vi "VST Streaming.vi"() -> ()   [LabVIEW 2021]
doc: "Demonstrates how to acquire I/Q data using the RF vector signal analyzer. The example shows how to configure NI-RFSA for continuous I/Q acquisition, how to set the carrier frequency and the I/Q rate, and how to fetch I/Q data. The dBm calculation is applied to I/Q magnitude to produce signal power and display it on the graph."
uses:
  Messaging/Write Message with Waveform.ctl
  RFSA/Support/RFSA Configuration.ctl
  Messaging/RFSA Message.ctl
  RFSG/Support/RFSG Configuration.ctl
  Messaging/RFSG Message.ctl
panel:
  in  "bandwidth":dbl(slide)=1000000.0 caption="Bandwidth" min=10000.0 max=200000000.0 step=1000000.0 scale=10000.0..200000000.0
  in  "freq.off":i32(slide)=2 caption="Frequency Offset" min=0 max=10000000 step=1000 scale=0.0..10000000.0 scale format="%.0pHz"
  in  "resolution":i64(slide)=1000 caption="Resolution" min=1000 max=100000 step=1000 scale=100000.0..1000.0
  in  "center.freq":dbl(slide)=4000000000.0 caption="Center Frequency" min=500000000.0 max=5500000000.0 step=500000000.0 scale=500000000.0..5500000000.0 scale format="%.1f"
  in  "pwr":dbl(slide)=-10.0 caption="Power" min=-60.0 max=0.0 step=1.0
  in  "rfsg.rsrc":refnum<k15>="5646VST" caption="RFSG Resource"
  in  "rfsa.rsrc":refnum<k15>="5646VST" caption="RFSA Resource"
  in  "start.rf":bool
  in  "stop.rf":bool
  in  "write?":bool
  in  "plot iq?":bool
  out "pred.acq.rate":dbl caption="Predicted Acquisition Rate" format="%#_4pB/s"
  out "pred.blk.size":dbl caption="Predicted Block Size" format="%#_4pB"
  in  "Clear Charts":bool
  out "Write to Disk Rate":dbl format="%#_4pB/s"
  out "Actual Execution Rate":dbl format="%#_4pB/s"
  out "Actual Acquisition Rate":dbl format="%#_4pB/s"
  out "Actual Block Size":i32 format="%.0pB"
  out "iq data":cluster{dbl[], dbl[]}(graph)
  # "200MHz"
  # "10kHz"
  # "10MHz"
  # "0Hz"
  # "1kHz"
  # "100kHz"
  # "5.5GHz"
  # "500MHz"
  # "0dB"
  # "-60dB"
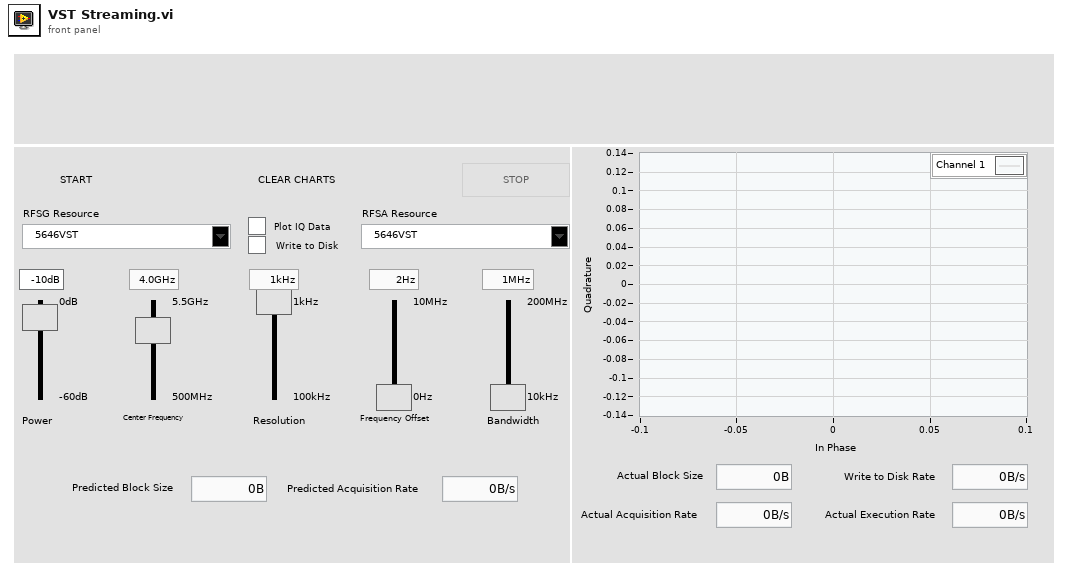
[diagram p1: front panel]
types:
  T1 = enum8{"Enabled", "Disabled", "Disabled and Grayed Out"}
  T2 = typedef "RFSG Configuration.ctl" = cluster{"rfsg ref":refnum<k15>, "freq off":i32, "wfm type":u16, "cent freq":dbl, "iq rate":dbl, "power":dbl, "msg":T3}
  T3 = typedef "RFSG Message.ctl" = enum16{"Trigger Ready", "Run RF", "Stop RF", "Exit"}
  T4 = typedef "RFSA Configuration.ctl" = cluster{"rfsa ref":refnum<k15>, "cent freq":dbl, "iq rate":dbl, "power":dbl, "N/block":i64, "msg":T5}
  T5 = typedef "RFSA Message.ctl" = enum16{"Trigger Ready", "Run RF", "Stop RF", "Exit"}
  T6 = typedef "Write Message with Waveform.ctl" = cluster{"wfm dat":waveform(cdb), "msg":enum16{"Close TDMS", "Initialize TDMS", "Write", "Exit"}}
  T7 = enum32{"invalid app kind", "Development System", "Run Time System", "Student Edition", "Embedded LabVIEW", "Evaluation", "Custom"}
  T8 = enum16{"Close TDMS", "Initialize TDMS", "Write", "Exit"}
  T9 = enum16{"open", "open or create", "create or replace", "create", "open (read-only)"}
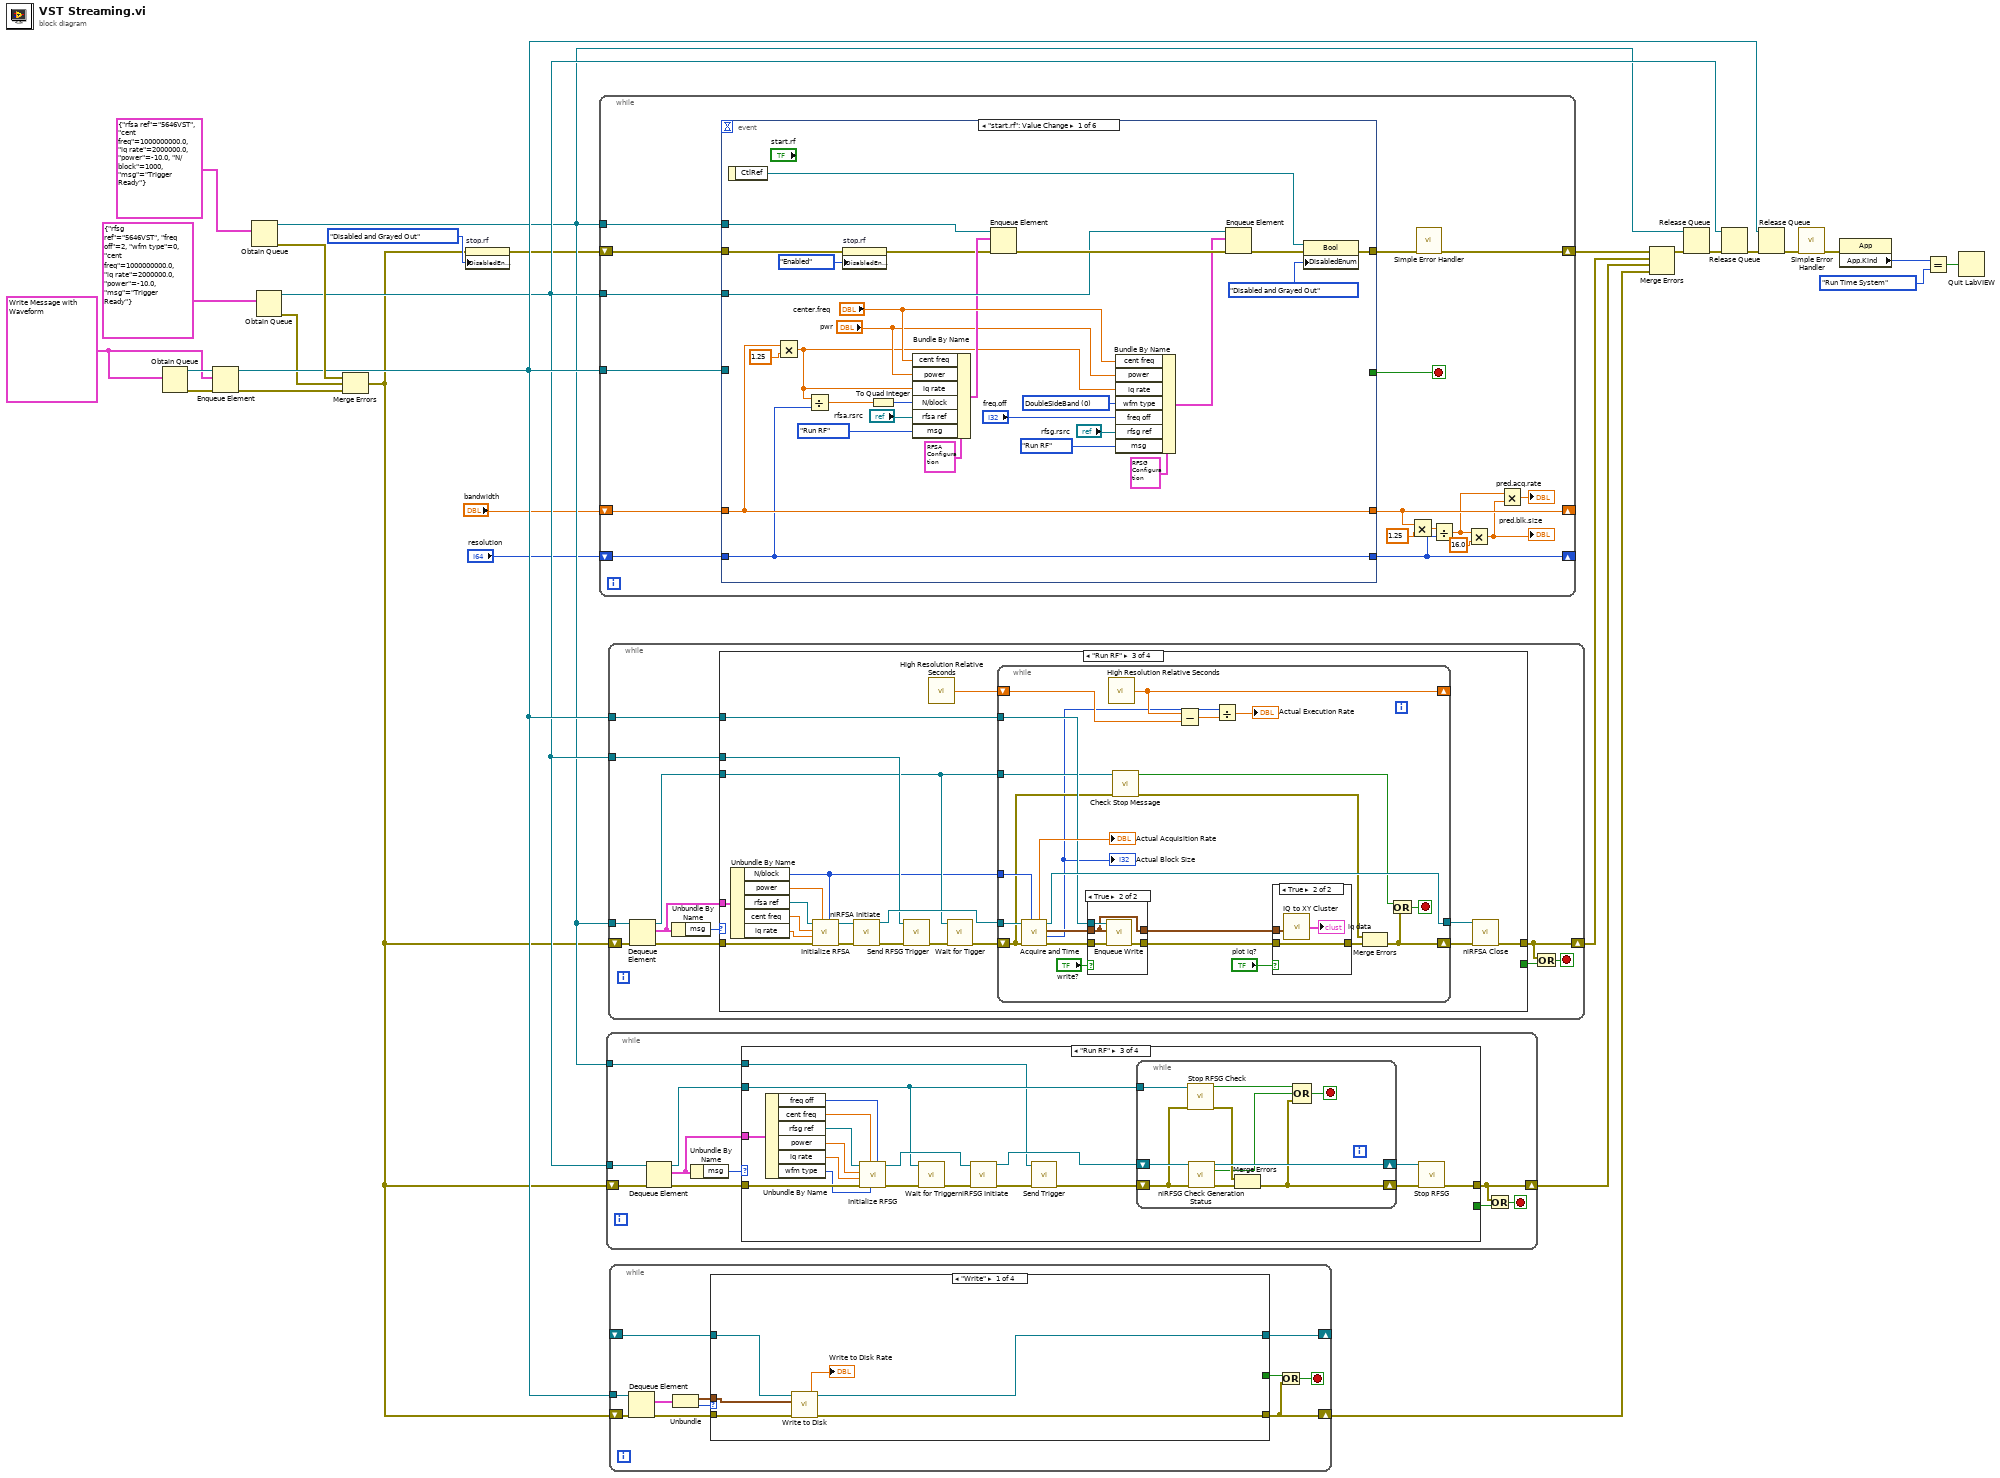
[diagram p0: block diagram]
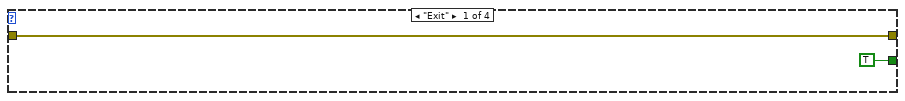
[diagram p2: hidden frame]
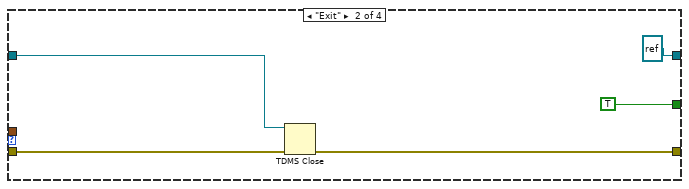
[diagram p5: hidden frame]
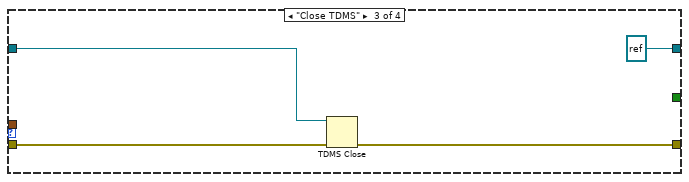
[diagram p6: hidden frame]
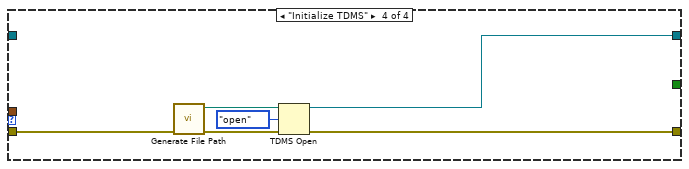
[diagram p7: hidden frame]
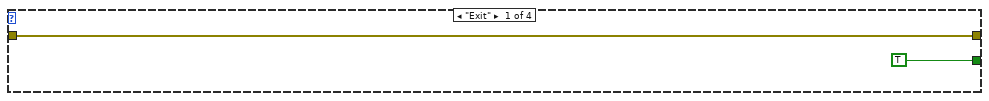
[diagram p8: hidden frame]
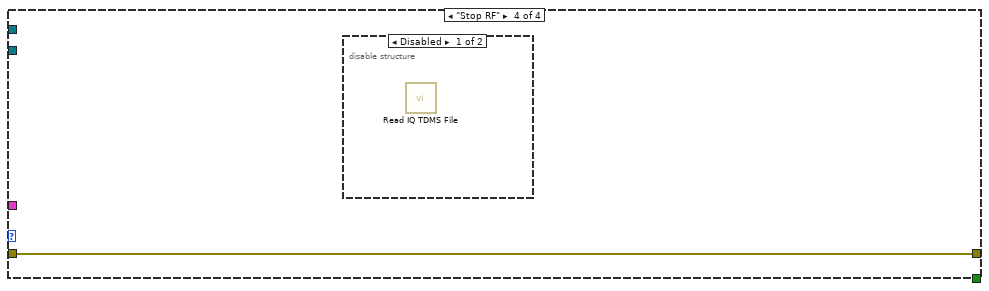
[diagram p12: hidden frame]
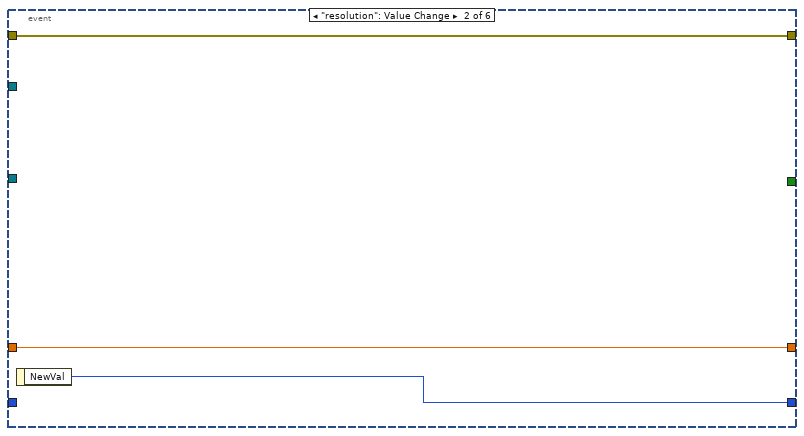
[diagram p14: hidden frame]
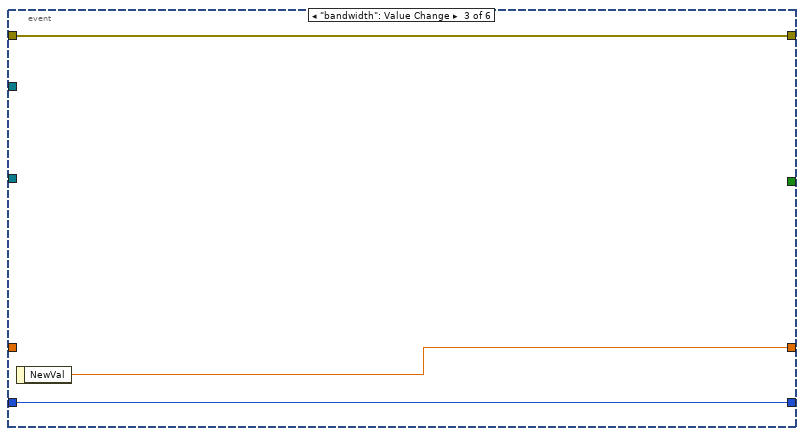
[diagram p15: hidden frame]
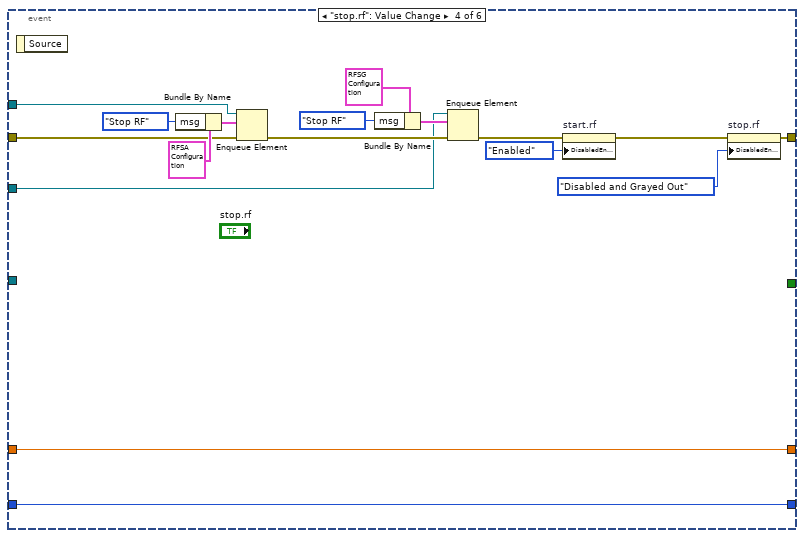
[diagram p16: hidden frame]
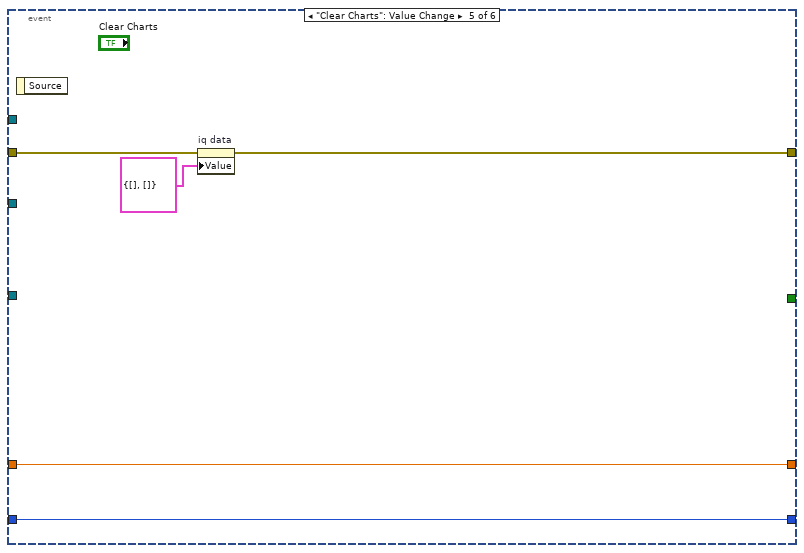
[diagram p17: hidden frame]
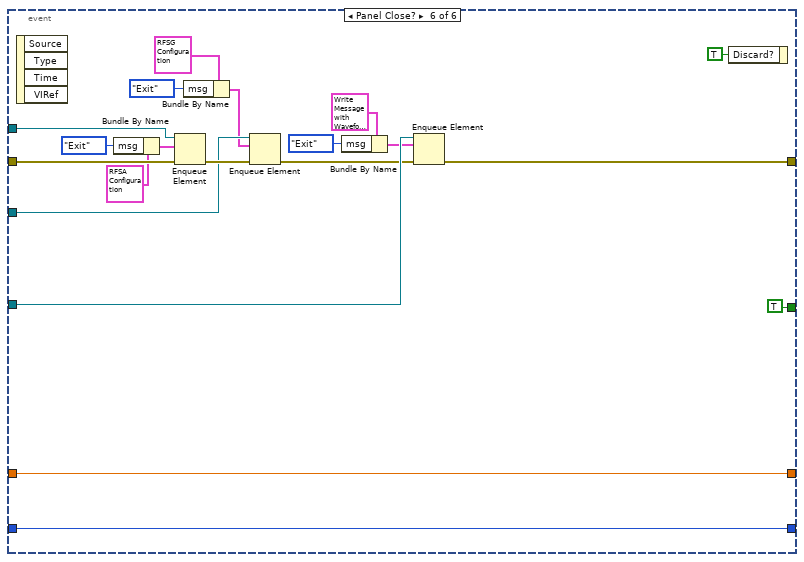
[diagram p18: hidden frame]
diagram:
  w18 = T6 {"wfm dat"={"t0"=timestamp(0 s since 1904-01-01), "dt"=0.0, "Y"=[]}, "msg"=enum."Initialize TDMS"}
  n1 = Obtain Queue(element data type=w18) -> (queue out=w24:refnum<queue>, error out=w25:errorcluster)  [unwired: 4 in, 1 out]
  n2 = Enqueue Element(queue=w24, element=w18, error in (no error)=w25) -> (queue out=w17:refnum<queue>, error out=w14:errorcluster)  [unwired: 1 in, 1 out]
  n3 = Obtain Queue(element data type=T4 {"rfsa ref"="5646VST", "cent freq"=1000000000.0, "iq rate"=2000000.0, "power"=-10.0, "N/block"=1000, "msg"=enum."Trigger Ready"}) -> (queue out=w7:refnum<queue>, error out=w19:errorcluster)  [unwired: 4 in, 1 out]
  n4 = Obtain Queue(element data type=T2 {"rfsg ref"="5646VST", "freq off"=2, "wfm type"=0, "cent freq"=1000000000.0, "iq rate"=2000000.0, "power"=-10.0, "msg"=enum."Trigger Ready"}) -> (queue out=w8:refnum<queue>, error out=w13:errorcluster)  [unwired: 4 in, 1 out]
  n5 = Merge Errors(w19, w13, w14) -> (w4:errorcluster)
  n6 = property on="stop.rf" class="Bool"(error in=w4, "DisabledEnum"=T1."Disabled and Grayed Out" ("Disabled")) -> (error out=w3:errorcluster)  [unwired: 1 in, 1 out]
  n7 = while {
    shift-right: [w32] -> w28
    shift-left: w3 -> [w44]
    tunnel: w7 -> [w45]
    tunnel: w17 -> [w43]
    tunnel: w8 -> [w42]
    shift-right: [w31] -> _
    shift-left: "bandwidth" -> [w39]
    shift-right: [w35] -> _
    shift-left: "resolution" -> [w38]
    stop <- w34 stop-if-true
    n8 = event shown="[0] \"start.rf\": Value Change" {
      selector: _ -> [_ _ _ _ _ _]
      dyn-events: _ -> [_ _ _ _ _ _]
      timeout: _ -> [_ _ _ _ _ _]
      tunnel: w45 -> [w73 _ _ w88 _ w120]
      tunnel: w44 -> [w52 w74 w77 w89 w101 w121]
      tunnel: [w71 w74 w77 w83 w100 w104] -> w33
      tunnel: [_ _ _ _ _ TRUE ("Exit")] -> w34
      tunnel: w43 -> [_ _ _ _ _ w118]
      tunnel: w42 -> [w66 _ _ w87 _ w108]
      tunnel: w39 -> [w47 w75 _ w80 w98 w103]
      tunnel: [w46 w76 w78 w81 w97 w102] -> w35
      tunnel: w38 -> [w46 _ w78 w81 w97 w102]
      tunnel: [w47 w75 w79 w80 w98 w103] -> w31
      event "start.rf": Value Change {
        w62 = u16 0 items=["DoubleSideBand", "LowerSideBand", "UpperSideBand"] ("Selected Waveform")
        n9 = event-data() -> ("CtlRef"=w70:refnum<vi>)  [unwired: 1 in]
        n10 = Multiply(x=w47, y=1.25) -> (x*y=w49:dbl)
        n11 = Divide(x=w49, y=w46) -> (x/y=w56:dbl)
        n12 = property on="stop.rf" class="Bool"(error in=w52, "DisabledEnum"=T1."Enabled" ("Disabled")) -> (error out=w51:errorcluster)  [unwired: 1 in, 1 out]
        n13 = To Quad Integer(1:w56) -> (0:w48:i64)
        n14 = Bundle By Name(cluster=T4 {"rfsa ref"="5646VST", "cent freq"=1000000000.0, "iq rate"=2000000.0, "power"=-10.0, "N/block"=1000, "msg"=enum."Trigger Ready"} ("element"), "cent freq"="center.freq", "power"="pwr", "iq rate"=w49, "N/block"=w48, "rfsa ref"="rfsa.rsrc", "msg"=RFSA_Message."Run RF") -> (w59:T4)
        n15 = Enqueue Element(queue=w73, element=w59, error in (no error)=w51) -> (error out=w68:errorcluster)  [unwired: 1 in, 2 out]
        n16 = Bundle By Name(cluster=T2 {"rfsg ref"="5646VST", "freq off"=2, "wfm type"=0, "cent freq"=1000000000.0, "iq rate"=2000000.0, "power"=-10.0, "msg"=enum."Trigger Ready"} ("element"), "cent freq"="center.freq", "power"="pwr", "iq rate"=w49, "wfm type"=w62, "freq off"="freq.off", "rfsg ref"="rfsg.rsrc", "msg"=RFSG_Message."Run RF") -> (w57:T2)
        n17 = Enqueue Element(queue=w66, element=w57, error in (no error)=w68) -> (error out=w67:errorcluster)  [unwired: 1 in, 2 out]
        n18 = property class="Bool"(reference=w70, error in=w67, "DisabledEnum"=T1."Disabled and Grayed Out" ("Disabled")) -> (error out=w71:errorcluster)  [unwired: 1 out]
      }
      event "resolution": Value Change {
        n19 = event-data() -> ("NewVal"=w76:i64)  [unwired: 1 in]
      }
      event "bandwidth": Value Change {
        n20 = event-data() -> ("NewVal"=w79:dbl)  [unwired: 1 in]
      }
      event "stop.rf": Value Change {
        n21 = event-data() -> ()  [unwired: 1 in, 1 out]
        n22 = Bundle By Name(cluster=T4 {"rfsa ref"="5646VST", "cent freq"=1000000000.0, "iq rate"=2000000.0, "power"=-10.0, "N/block"=1000, "msg"=enum."Trigger Ready"} ("element"), "msg"=RFSA_Message."Stop RF") -> (w94:T4)
        n23 = Enqueue Element(queue=w88, element=w94, error in (no error)=w89) -> (error out=w93:errorcluster)  [unwired: 1 in, 2 out]
        n24 = Bundle By Name(cluster=T2 {"rfsg ref"="5646VST", "freq off"=2, "wfm type"=0, "cent freq"=1000000000.0, "iq rate"=2000000.0, "power"=-10.0, "msg"=enum."Trigger Ready"} ("element"), "msg"=RFSG_Message."Stop RF") -> (w90:T2)
        n25 = Enqueue Element(queue=w87, element=w90, error in (no error)=w93) -> (error out=w86:errorcluster)  [unwired: 1 in, 2 out]
        n26 = property on="start.rf" class="Bool"(error in=w86, "DisabledEnum"=T1."Enabled" ("Disabled")) -> (error out=w84:errorcluster)  [unwired: 1 in, 1 out]
        n27 = property on="stop.rf" class="Bool"(error in=w84, "DisabledEnum"=T1."Disabled and Grayed Out" ("Disabled")) -> (error out=w83:errorcluster)  [unwired: 1 in, 1 out]
      }
      event "Clear Charts": Value Change {
        n28 = event-data() -> ()  [unwired: 1 in, 1 out]
        n29 = property on="iq data" class="XYGraph (strict)"(error in=w101, "Value"=cluster{dbl[], dbl[]} {[], []} ("iq data")) -> (error out=w100:errorcluster)  [unwired: 1 in, 1 out]
      }
      event Panel Close? {
        n30 = event-data() -> ()  [unwired: 1 in, 4 out]
        n31 = Bundle By Name(cluster=T4 {"rfsa ref"="5646VST", "cent freq"=1000000000.0, "iq rate"=2000000.0, "power"=-10.0, "N/block"=1000, "msg"=enum."Trigger Ready"} ("element"), "msg"=RFSA_Message."Exit") -> (w111:T4)
        n32 = Enqueue Element(queue=w120, element=w111, error in (no error)=w121) -> (error out=w110:errorcluster)  [unwired: 1 in, 2 out]
        n33 = Bundle By Name(cluster=T2 {"rfsg ref"="5646VST", "freq off"=2, "wfm type"=0, "cent freq"=1000000000.0, "iq rate"=2000000.0, "power"=-10.0, "msg"=enum."Trigger Ready"} ("element"), "msg"=RFSG_Message."Exit") -> (w105:T2)
        n34 = Enqueue Element(queue=w108, element=w105, error in (no error)=w110) -> (error out=w109:errorcluster)  [unwired: 1 in, 2 out]
        n35 = Bundle By Name(cluster=T6 {"wfm dat"={"t0"=timestamp(0 s since 1904-01-01), "dt"=0.0, "Y"=[]}, "msg"=enum."Exit"} ("element"), "msg"=T8."Exit") -> (w115:T6)
        n36 = Enqueue Element(queue=w118, element=w115, error in (no error)=w109) -> (error out=w104:errorcluster)  [unwired: 1 in, 2 out]
        n37 = event-data("Discard?"=TRUE) -> ()  [unwired: 1 in, 1 out]
      }
    }
    n38 = Multiply(x=w31, y=1.25) -> (x*y=w36:dbl)
    n39 = call <vilib>:"Simple Error Handler.vi"("error in (no error)"=w33) -> ("error out"=w32:errorcluster)  [unwired: 4 in, 4 out]
    n40 = Divide(x=w36, y=w35) -> (x/y=w29:dbl)
    n41 = Multiply(x=w29, y=16.0) -> (x*y=w30:dbl)
    "pred.blk.size" <- w30
    n42 = Multiply(x=w29, y=w30) -> (x*y=→"pred.acq.rate":dbl)
  }
  n43 = while {
    shift-right: [w127] -> w9
    shift-left: w4 -> [w130]
    tunnel: w8 -> [w126]
    tunnel: w7 -> [w122]
    stop <- w129 stop-if-true
    n44 = Dequeue Element(queue=w126, error in (no error)=w130) -> (queue out=w123:refnum<queue>, element=w125:T2, error out=w131:errorcluster)  [unwired: 1 in, 1 out]
    n45 = Unbundle By Name(w125) -> ("msg"=w124:T3)
    n46 = case shown="\"Run RF\"" w124 {
      tunnel: w131 -> [w132 w134 w153 w164]
      tunnel: [w132 w134 w148 w164] -> w127
      tunnel: [TRUE ("x") _ _ _] -> w128
      tunnel: w125 -> [_ _ w147 _]
      tunnel: w123 -> [_ _ w138 _]
      tunnel: w122 -> [_ _ w135 _]
      frame "Exit" {
      }
      frame "Trigger Ready" {
      }
      frame "Run RF" {
        n47 = Unbundle By Name(w147) -> ("freq off"=w141:i32, "cent freq"=w142:dbl, "rfsg ref"=w143:refnum<k15>, "power"=w144:dbl, "iq rate"=w145:dbl, "wfm type"=w146:u16)
        n48 = call "Initialize RFSG.vi"("Frequency Offset"=w141, "Selected Waveform"=w146, "Center Frequency"=w142, "error in (no error)"=w153, "IQ Rate"=w145, "Power Level"=w144, "RFSG Reference In"=w143) -> ("error out"=w140:errorcluster, "RFSG Reference Out"=w152:refnum<k15>)  [unwired: 1 in, 2 out]
        n49 = call "Wait for Trigger.vi"("error in (no error)"=w140, "rfsg queue"=w138) -> ("error out"=w139:errorcluster)  [unwired: 8 in, 1 out]
        n50 = call <instrlib>:"niRFSG Initiate.vi"("instrument handle"=w152, "error in"=w139) -> ("instrument handle out"=w151:refnum<k15>, "error out"=w137:errorcluster)  [unwired: 12 in]
        n51 = call "Send Trigger.vi"("error in (no error)"=w137, "rfsa queue"=w135) -> ("error out"=w136:errorcluster)  [unwired: 9 in]
        n52 = while {
          shift-right: [w157] -> w150
          shift-left: w136 -> [w161]
          shift-right: [w162] -> w149
          shift-left: w151 -> [w163]
          tunnel: w138 -> [w160]
          stop <- w154 stop-if-true
          n53 = call "Stop RFSG Check.vi"("error in (no error)"=w161, "rfsg queue"=w160) -> ("error out"=w158:errorcluster, "stop?"=w156:bool)  [unwired: 8 in]
          n54 = call <instrlib>:"niRFSG Check Generation Status.vi"("instrument handle"=w163, "error in"=w161) -> ("instrument handle out"=w162:refnum<k15>, "done?"=w155:bool, "error out"=w159:errorcluster)  [unwired: 11 in]
          n55 = Merge Errors(w158, w159) -> (w157:errorcluster)
          n56 = Compound Arithmetic op=OR(w156, w155, w157) -> (w154:bool)
        }
        n57 = call "Stop RFSG.vi"("error in (no error)"=w150, "RFSG Reference In"=w149) -> ("error out"=w148:errorcluster)  [unwired: 9 in]
      }
      frame "Stop RF" {
      }
    }
    n58 = Or(x=w127, y=w128) -> (x .or. y?=w129:bool)
  }
  n59 = while {
    tunnel: w7 -> [w172]
    shift-right: [w170] -> w26
    shift-left: w4 -> [w174]
    tunnel: w17 -> [w169]
    tunnel: w8 -> [w165]
    stop <- w173 stop-if-true
    n60 = Dequeue Element(queue=w172, error in (no error)=w174) -> (queue out=w166:refnum<queue>, element=w168:T4, error out=w175:errorcluster)  [unwired: 1 in, 1 out]
    n61 = Unbundle By Name(w168) -> ("msg"=w167:T5)
    n62 = case shown="\"Run RF\"" w167 {
      tunnel: w175 -> [w176 w178 w198 w232]
      tunnel: [w176 w178 w191 w232] -> w170
      tunnel: [TRUE ("x") _ _ _] -> w171
      tunnel: w169 -> [_ _ w192 _]
      tunnel: w168 -> [_ _ w190 _]
      tunnel: w166 -> [_ _ w181 _]
      tunnel: w165 -> [_ _ w184 _]
      frame "Exit" {
      }
      frame "Trigger Ready" {
      }
      frame "Run RF" {
        n63 = Unbundle By Name(w190) -> ("N/block"=w180:i64, "power"=w186:dbl, "rfsa ref"=w187:refnum<k15>, "cent freq"=w188:dbl, "iq rate"=w189:dbl)
        n64 = call "Initialize RFSA.vi"("N/block"=w180, "Reference Level"=w186, "error in (no error)"=w198, "IQ Rate"=w189, "Carrier Frequency"=w188, "RFSA Reference In"=w187) -> ("error out"=w197:errorcluster, "RFSA Reference Out"=w196:refnum<k15>)  [unwired: 4 in]
        n65 = call <instrlib>:"niRFSA Initiate.vi"("instrument handle"=w196, "error in"=w197) -> ("instrument handle out"=w195:refnum<k15>, "error out"=w185:errorcluster)  [unwired: 12 in]
        n66 = call "Send RFSG Trigger.vi"("error in (no error)"=w185, "rfsg queue"=w184) -> ("error out"=w183:errorcluster)  [unwired: 9 in]
        n67 = call <vilib>:"High Resolution Relative Seconds.vi"() -> ("relative seconds"=w179:dbl)
        n68 = call "Wait for Tigger.vi"("error in (no error)"=w183, "rfsa queue"=w181) -> ("error out"=w182:errorcluster)  [unwired: 8 in, 1 out]
        n69 = while {
          shift-right: [w206] -> w194
          shift-left: w182 -> [w211]
          tunnel: [w221] -> w193
          tunnel: w195 -> [w220]
          tunnel: w180 -> [w219]
          tunnel: w192 -> [w217]
          tunnel: w181 -> [w212]
          shift-right: [w202] -> _
          shift-left: w179 -> [w203]
          stop <- w210 stop-if-true
          n70 = call "Acquire and Time.vi"("samples per block"=w219, "error in (no error)"=w211, "RFSA Reference In"=w220) -> ("error out"=w204:errorcluster, "bytes"=w201:i32, "data"=w205:waveform(cdb), "RFSA Reference Out"=w221:refnum<k15>, "DAQ B/sec"=→"Actual Acquisition Rate":dbl)  [unwired: 4 in]
          "Actual Block Size" <- w201
          n71 = case shown="True" "write?" {
            tunnel: w204 -> [w227 w231]
            tunnel: [w227 w230] -> w213
            tunnel: w217 -> [_ w229]
            tunnel: w205 -> [w226 w228]
            tunnel: [w226 w228] -> w215
            frame False {
            }
            frame True {
              n72 = call "Enqueue Write.vi"("error in (no error)"=w231, "data"=w228, "disk queue"=w229) -> ("error out"=w230:errorcluster)  [unwired: 8 in]
            }
          }
          n73 = call <vilib>:"High Resolution Relative Seconds.vi"() -> ("relative seconds"=w202:dbl)
          n74 = call "Check Stop Message.vi"("error in (no error)"=w211, "rfsa queue"=w212) -> ("error out"=w207:errorcluster, "stop?"=w209:bool)  [unwired: 8 in]
          n75 = Subtract(x=w202, y=w203) -> (x-y=w200:dbl)
          n76 = Divide(x=w201, y=w200) -> (x/y=→"Actual Execution Rate":dbl)
          n77 = case shown="True" "plot iq?" {
            tunnel: w215 -> [_ w225]
            tunnel: w213 -> [w222 w223]
            tunnel: [w222 w223] -> w208
            frame False {
            }
            frame True {
              n78 = call "IQ to XY Cluster.vi"("wfm data"=w225) -> ("xy cluster"=→"iq data":cluster{"Array":dbl[], "Array":dbl[]})
            }
          }
          n79 = Merge Errors(w207, w208) -> (w206:errorcluster)
          n80 = Or(x=w209, y=w206) -> (x .or. y?=w210:bool)
        }
        n81 = call <instrlib>:"niRFSA Close.vi"("instrument handle"=w193, "error in"=w194) -> ("error out"=w191:errorcluster)  [unwired: 13 in]
      }
      frame "Stop RF" {
        n82 = disable-structure shown="Disabled" {
          frame Disabled {
            n83 = call "Read IQ TDMS File.vi"() -> ()  [unwired: 9 in, 3 out]
          }
          frame Enabled {
          }
        }
      }
    }
    n84 = Or(x=w170, y=w171) -> (x .or. y?=w173:bool)
  }
  n85 = while {
    shift-right: [w239] -> w10
    shift-left: w4 -> [w242]
    tunnel: w17 -> [w238]
    shift-right: [w236] -> _
    shift-left: _ -> [w237]
    stop <- w241 stop-if-true
    n86 = Dequeue Element(queue=w238, error in (no error)=w242) -> (element=w235:T6, error out=w243:errorcluster)  [unwired: 1 in, 2 out]
    n87 = Unbundle(w235) -> ("wfm dat"=w233:waveform(cdb), "msg"=w234:T8)
    n88 = case shown="\"Write\"" w234 {
      tunnel: w243 -> [w245 w253 w258 w261]
      tunnel: [w247 w252 w257 w263] -> w239
      tunnel: [_ TRUE ("x") _ _] -> w240
      tunnel: w237 -> [w249 w251 w256 _]
      tunnel: [w248 refnum<k34> refnum ("tdms file out") refnum<k34> refnum ("tdms file out") w262] -> w236
      tunnel: w233 -> [w244 _ _ _]
      frame "Write" {
        n89 = call "Write to Disk.vi"("error in (no error)"=w245, "wfm dat in"=w244, "tdms file"=w249) -> ("error out"=w247:errorcluster, "tdms file out"=w248:refnum<k34>, "Bytes Analyzed per Second"=→"Write to Disk Rate":dbl)  [unwired: 5 in, 1 out]
      }
      frame "Exit" {
        n90 = TDMS Close(8:w253, 11:w251) -> (0:w252:errorcluster)  [unwired: 1 out]
      }
      frame "Close TDMS" {
        n91 = TDMS Close(8:w258, 11:w256) -> (0:w257:errorcluster)  [unwired: 1 out]
      }
      frame "Initialize TDMS" {
        n92 = call "Generate File Path.vi"("error in (no error)"=w261) -> ("error out"=w260:errorcluster, "file path"=w259:path)  [unwired: 9 in]
        n93 = TDMS Open(8:w260, 10:T9."open" ("operation (0:open)"), 11:w259) -> (0:w263:errorcluster, 3:w262:refnum<k34>)  [unwired: 4 in]
      }
    }
    n94 = Or(x=w240, y=w239) -> (x .or. y?=w241:bool)
  }
  n95 = Merge Errors(w28, w26, w9, w10) -> (w27:errorcluster)
  n96 = Release Queue(queue=w7, error in (no error)=w27) -> (error out=w12:errorcluster)  [unwired: 1 in, 2 out]
  n97 = Release Queue(queue=w8, error in (no error)=w12) -> (error out=w11:errorcluster)  [unwired: 1 in, 2 out]
  n98 = Release Queue(queue=w17, error in (no error)=w11) -> (error out=w6:errorcluster)  [unwired: 1 in, 2 out]
  n99 = call <vilib>:"Simple Error Handler.vi"("error in (no error)"=w6) -> ("error out"=w23:errorcluster)  [unwired: 4 in, 4 out]
  n100 = property class="App"(error in=w23) -> ("App.Kind"=w22:T7)  [unwired: 1 in, 2 out]
  n101 = Equal?(x=w22, y=T7."Run Time System") -> (x = y?=w20:bool)
  n102 = Quit LabVIEW(quit? (T)=w20) -> ()
